vi "Periodic Tasks.vi"(8 "error in":errorcluster) -> ()   [LabVIEW 2020]
doc: "This VI runs in parallel to other tasks. It can contain as many user-defined periodic loops as you need. These can carry out PID or other sorts of timed response."
uses:
  <vilib>/Rock Robotics/WPI/Utilities/WPI_GetSetVariantRefNum.vi
  <vilib>/addons/control/pid/pid.llb/PID (DBL).vi
  <vilib>/addons/control/pid/NI_PID_pid.lvlib
panel:
  in  "output range":cluster{"output high":dbl, "output low":dbl}={"output high"=100.0, "output low"=-100.0} {"output low" format="%.2f"; "output high" format="%.2f"}
  in  "Output 2 PID gains":T1={"proportional gain (Kc)"=1.0, "integral time (Ti, min)"=0.01, "derivative time (Td, min)"=0.0} {"derivative time (Td, min)" format="%.3f"; "integral time (Ti, min)" format="%.3f"; "proportional gain (Kc)" format="%.3f"}
  in  "Output 2 RPM Setpoint":dbl
  in  "Output 2 Use PID":bool
  out "Shooter Stopped":bool
  in  "Output 2 Use limits":bool
  in  "Output 1 Use limits":bool
  out "Shooter Speed":dbl
  in  "Enabled 2":bool
  in  "Output 2":dbl(slide) scale=-1.0..1.0
  in  "Enabled":bool
  in  "Output":dbl(slide) scale=-1.0..1.0
  # "20 degrees angle,\n0.6 speed = 5 ft - 2400 rpm\n0.8 speed = 9 feet - 3000 rpm\nBattery at 11.8 volts"
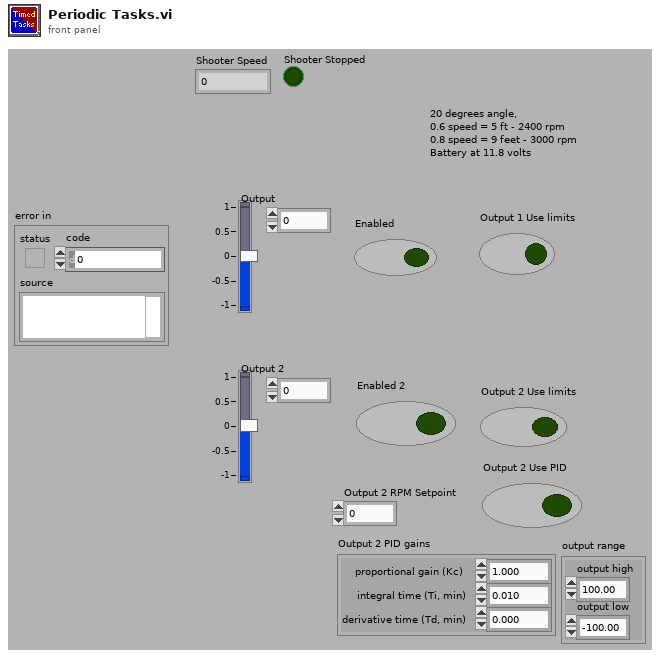
[diagram p1: front panel]
types:
  T1 = cluster{"proportional gain (Kc)":dbl, "integral time (Ti, min)":dbl, "derivative time (Td, min)":dbl}
  T2 = typedef "WPI_JoystickDevRef.ctl" = cluster{"Device":T3}
  T3 = typedef "WPI_JoystickDeviceEnum.ctl" = enum16{"USB 0", "USB 1", "USB 2", "USB 3", "USB 4", "USB 5"}
  T4 = typedef "WPI_MotorControlDeviceRef.ctl" = cluster{"DeviceStatus":errorcluster, "Type":T5, "PWM":cluster{"PWM Channel":T6, "DeadBand":T7}, "CAN":cluster{"Device Number":u8, "SetOutput VI Ref":variant, "GetOutput VI Ref":variant, "Enable VI Ref":variant, "Disable VI Ref":variant, "Data":variant}, "Invert":bool, "DIO PWM":cluster{"PWM \"Enable\" Channel":T6, "DIOChannel":T8, "PWM Rate":dbl}}
  T5 = typedef "WPI_MotorControlType.ctl" = enum16{"PWM", "CAN", "DIO PWM"}
  T6 = typedef "FPGA_DIOPWMChannel.ctl" = enum8{"PWM 0", "PWM 1", "PWM 2", "PWM 3", "PWM 4", "PWM 5", "PWM 6", "PWM 7", "PWM 8", "PWM 9", "PWM MXP 0", "PWM MXP 1", "PWM MXP 2", "PWM MXP 3", "PWM MXP 4", "PWM MXP 5", "PWM MXP 6", "PWM MXP 7", "PWM MXP 8", "PWM MXP 9", "Invalid"}
  T7 = typedef "WPI_PWMDeadband.ctl" = cluster{"Name":string, "maxPositivePwm":i32, "minPositivePwm":i32, "centerPwm":i32, "maxNegativePwm":i32, "minNegativePwm":i32, "angularRange":u16}
  T8 = typedef "FPGA_DIOChannel.ctl" = enum8{"DIO 0", "DIO 1", "DIO 2", "DIO 3", "DIO 4", "DIO 5", "DIO 6", "DIO 7", "DIO 8", "DIO 9", "DIO MXP 0", "DIO MXP 1", "DIO MXP 2", "DIO MXP 3", "DIO MXP 4", "DIO MXP 5", "DIO MXP 6", "DIO MXP 7", "DIO MXP 8", "DIO MXP 9", "DIO MXP 10", "DIO MXP 11", "DIO MXP 12", "DIO MXP 13", "DIO MXP 14", "DIO MXP 15", "SPI Port CS1", "SPI Port CS2", "SPI Port CS3", "SPI Port MISO", "SPI Port MOSI", "Invalid"}
  T9 = typedef "WPI_EncoderDevRef.ctl" = cluster{"DevStatus":errorcluster, "EncoderIndex":T10, "CounterIndex":T11, "DistancePerCount":dbl, "Decoding Type":T12}
  T10 = typedef "FPGA_EncoderIdx.ctl" = enum8{"Enc 0", "Enc 1", "Enc 2", "Enc 3", "Enc 4", "Enc 5", "Enc 6", "Enc 7", "Invalid"}
  T11 = typedef "FPGA_CounterCtrSystemIndex.ctl" = enum8{"Ctr 0", "Ctr 1", "Ctr 2", "Ctr 3", "Ctr 4", "Ctr 5", "Ctr 6", "Ctr 7", "Invalid"}
  T12 = typedef "WPI_EncoderType.ctl" = enum16{"1x", "2x", "4x"}
  T13 = typedef "WPI_SwitchDevRef.ctl" = cluster{"DevStatus":errorcluster, "DIO Channel":T8, "CntIndex":T11, "Normally Closed":bool}
  T14 = cluster{"JoystickDevRef":T2, "MotorControlDevRef":T4, "MotorControlDevRef":T4, "EncoderDevRef":T9, "SwitchDevRef":T13, "SwitchDevRef":T13}
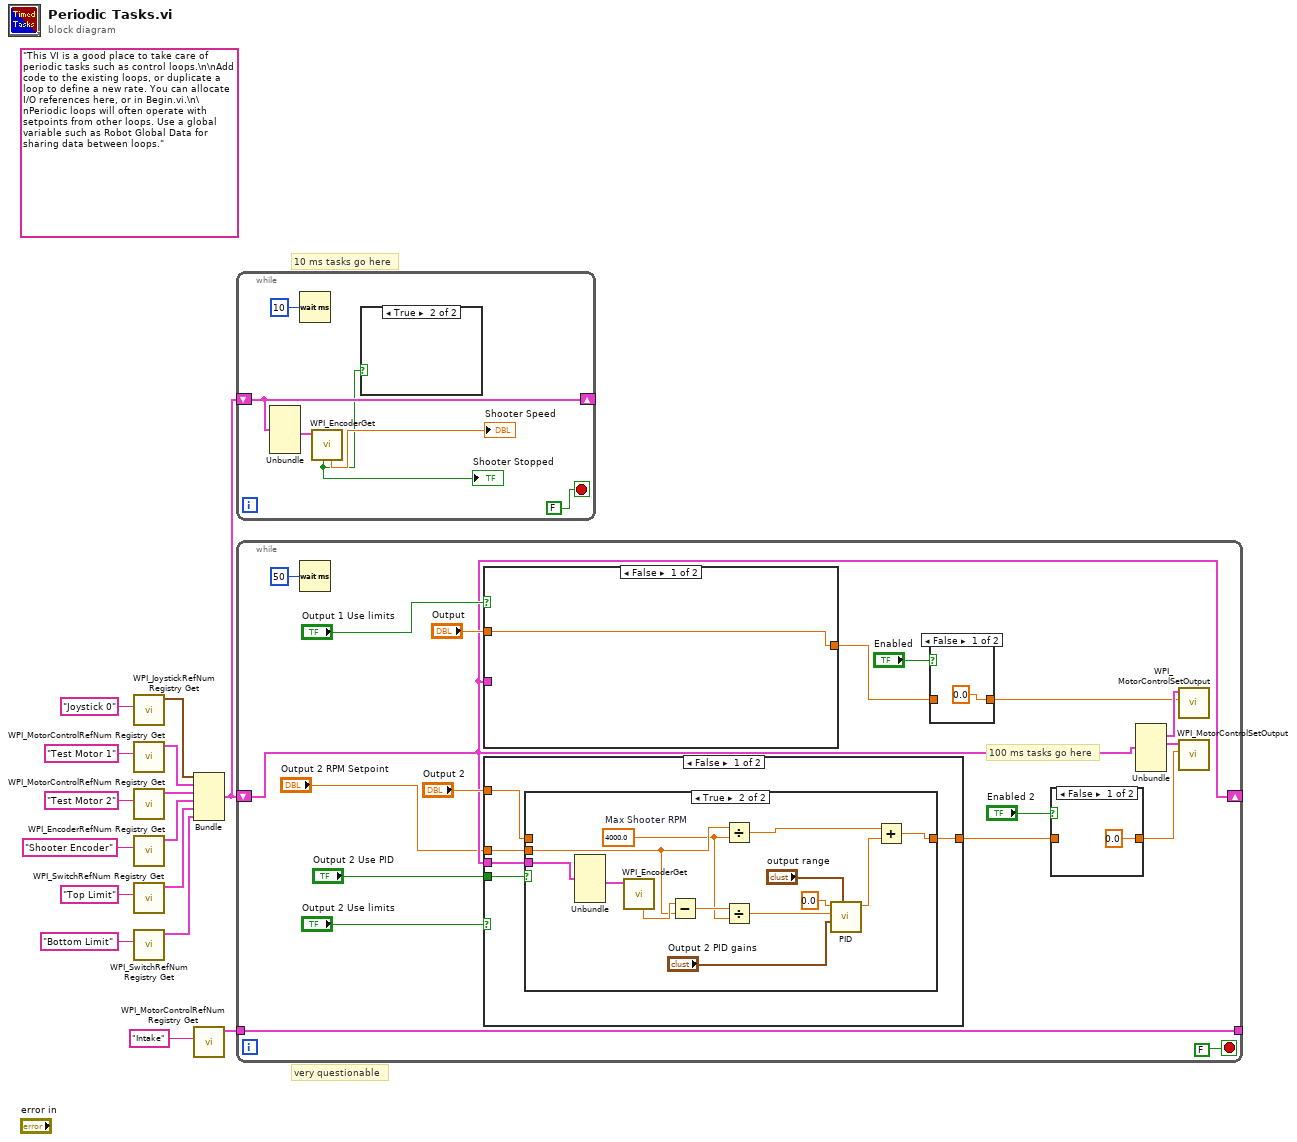
[diagram p0: block diagram]
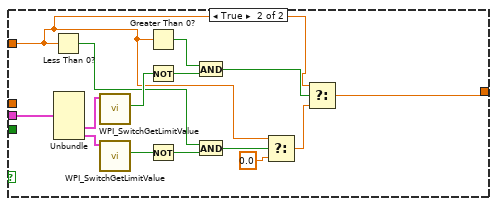
[diagram p5: hidden frame]
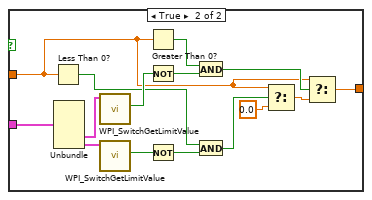
[diagram p6: hidden frame]
diagram:
  (unwired) "This VI is a good place to take care of periodic tasks such as control loops.\n\nAdd code to the existing loops, or duplicate a loop to define a new rate. You can allocate I/O references here, or in Begin.vi.\n\nPeriodic loops will often operate with setpoints from other loops. Use a global variable such as Robot Global Data for sharing data between loops."
  # "very questionable"
  # "10 ms tasks go here"
  n1 = call <vilib>:"WPI_JoystickRefNum Registry Get.vi"("refnum name"="Joystick 0") -> ("JoystickDevRef"=w14:T2)  [unwired: 1 in, 9 out]
  n2 = call <vilib>:"WPI_MotorControlRefNum Registry Get.vi"("refnum name"="Test Motor 1") -> ("MotorControlDevRef"=w11:T4)  [unwired: 9 in, 1 out]
  n3 = call <vilib>:"WPI_MotorControlRefNum Registry Get.vi"("refnum name"="Test Motor 2") -> ("MotorControlDevRef"=w9:T4)  [unwired: 9 in, 1 out]
  n4 = call <vilib>:"WPI_EncoderRefNum Registry Get.vi"("refnum name"="Shooter Encoder") -> ("EncoderDevRef"=w1:T9)  [unwired: 9 in, 1 out]
  n5 = call <vilib>:"WPI_SwitchRefNum Registry Get.vi"("refnum name"="Top Limit") -> ("SwitchDevRef"=w7:T13)  [unwired: 9 in, 1 out]
  n6 = call <vilib>:"WPI_SwitchRefNum Registry Get.vi"("refnum name"="Bottom Limit") -> ("SwitchDevRef"=w4:T13)  [unwired: 9 in, 1 out]
  n7 = Bundle("JoystickDevRef"=w14, "MotorControlDevRef"=w11, "MotorControlDevRef"=w9, "EncoderDevRef"=w1, "SwitchDevRef"=w7, "SwitchDevRef"=w4) -> (w13:T14)  [unwired: 1 out]
  n8 = call <vilib>:"WPI_MotorControlRefNum Registry Get.vi"("refnum name"="Intake") -> ("MotorControlDevRef"=w2:T4)  [unwired: 9 in, 1 out]
  n9 = while {
    shift-right: [w19] -> _
    shift-left: w13 -> [w19]
    stop <- FALSE stop-if-true
    n10 = Unbundle(w19) -> ("EncoderDevRef"=w17:T9)  [unwired: 5 out]
    n11 = Wait (ms)(milliseconds to wait=u32 10) -> ()  [unwired: 1 out]
    n12 = call <vilib>:"WPI_EncoderGet.vi"("EncoderDevRef"=w17) -> ("Rate"=→"Shooter Speed":dbl, "Stopped"=w16:bool)  [unwired: 5 in, 4 out]
    "Shooter Stopped" <- w16
    n13 = case shown="True" w16 {
      frame False {
      }
      frame True {
      }
    }
  }
  n14 = while {
    shift-right: [w33] -> _
    shift-left: w13 -> [w33]
    tunnel: [w25] -> _
    tunnel: w2 -> [w25]
    stop <- FALSE stop-if-true
    # "100 ms tasks go here"
    n15 = Wait (ms)(milliseconds to wait=u32 50) -> ()  [unwired: 1 out]
    n16 = case shown="False" "Output 1 Use limits" {
      tunnel: "Output" -> [w78 w80]
      tunnel: [w78 w87] -> w30
      tunnel: w33 -> [_ w93]
      frame False {
      }
      frame True {
        n17 = Less Than 0?(x=w80) -> (x < 0?=w86:bool)
        n18 = Unbundle(w93) -> ("SwitchDevRef"=w92:T13, "SwitchDevRef"=w81:T13)  [unwired: 4 out]
        n19 = call <vilib>:"WPI_SwitchGetLimitValue.vi"("SwitchDevRef"=w92) -> ("Switch Pressed"=w90:bool)  [unwired: 8 in, 2 out]
        n20 = call <vilib>:"WPI_SwitchGetLimitValue.vi"("SwitchDevRef"=w81) -> ("Switch Pressed"=w82:bool)  [unwired: 8 in, 2 out]
        n21 = Greater Than 0?(x=w80) -> (x > 0?=w91:bool)
        n22 = Not(x=w90) -> (.not. x?=w89:bool)
        n23 = Not(x=w82) -> (.not. x?=w85:bool)
        n24 = And(x=w91, y=w89) -> (x .and. y?=w88:bool)
        n25 = And(x=w86, y=w85) -> (x .and. y?=w84:bool)
        n26 = Select(t=w80, s=w84, f=0.0) -> (s? t:f=w79:dbl)
        n27 = Select(t=w80, s=w88, f=w79) -> (s? t:f=w87:dbl)
      }
    }
    n28 = case shown="False" "Output 2 Use limits" {
      tunnel: "Output 2" -> [w45 w64]
      tunnel: [w46 w71] -> w28
      tunnel: w33 -> [w44 w77]
      tunnel: "Output 2 Use PID" -> [w48 _]
      tunnel: "Output 2 RPM Setpoint" -> [w47 _]
      frame False {
        n29 = case shown="True" w48 {
          tunnel: w47 -> [_ w53]
          tunnel: [w49 w59] -> w46
          tunnel: w45 -> [w49 _]
          tunnel: w44 -> [_ w62]
          frame False {
          }
          frame True {
            w52 = 4000.0  # Max Shooter RPM
            n30 = Unbundle(w62) -> ("EncoderDevRef"=w61:T9)  [unwired: 5 out]
            n31 = call <vilib>:"WPI_EncoderGet.vi"("EncoderDevRef"=w61) -> ("Rate"=w56:dbl)  [unwired: 5 in, 5 out]
            n32 = Subtract(x=w56, y=w53) -> (x-y=w55:dbl)
            n33 = Divide(x=w53, y=w52) -> (x/y=w51:dbl)
            n34 = Divide(x=w55, y=w52) -> (x/y=w54:dbl)
            n35 = call-poly <vilib>:"PID.vi"("output range"="output range", "PID gains"="Output 2 PID gains", "process variable"=w54, "setpoint"=0.0) -> ("output"=w58:dbl)  [unwired: 6 in, 1 out]
            n36 = Add(x=w51, y=w58) -> (x+y=w59:dbl)
          }
        }
      }
      frame True {
        n37 = Less Than 0?(x=w64) -> (x < 0?=w70:bool)
        n38 = Unbundle(w77) -> ("SwitchDevRef"=w76:T13, "SwitchDevRef"=w65:T13)  [unwired: 4 out]
        n39 = call <vilib>:"WPI_SwitchGetLimitValue.vi"("SwitchDevRef"=w76) -> ("Switch Pressed"=w74:bool)  [unwired: 8 in, 2 out]
        n40 = call <vilib>:"WPI_SwitchGetLimitValue.vi"("SwitchDevRef"=w65) -> ("Switch Pressed"=w66:bool)  [unwired: 8 in, 2 out]
        n41 = Greater Than 0?(x=w64) -> (x > 0?=w75:bool)
        n42 = Not(x=w74) -> (.not. x?=w73:bool)
        n43 = Not(x=w66) -> (.not. x?=w69:bool)
        n44 = And(x=w75, y=w73) -> (x .and. y?=w72:bool)
        n45 = And(x=w70, y=w69) -> (x .and. y?=w68:bool)
        n46 = Select(t=w64, s=w68, f=0.0) -> (s? t:f=w63:dbl)
        n47 = Select(t=w64, s=w72, f=w63) -> (s? t:f=w71:dbl)
      }
    }
    n48 = case shown="False" "Enabled" {
      tunnel: w30 -> [_ w43]
      tunnel: [0.0 ("f") w43] -> w29
      frame False {
      }
      frame True {
      }
    }
    n49 = case shown="False" "Enabled 2" {
      tunnel: [0.0 ("Output") w41] -> w27
      tunnel: w28 -> [_ w41]
      frame False {
      }
      frame True {
      }
    }
    n50 = Unbundle(w33) -> ("MotorControlDevRef"=w37:T4, "MotorControlDevRef"=w36:T4)  [unwired: 4 out]
    n51 = call <vilib>:"WPI_MotorControlSetOutput.vi"("Output"=w29, "MotorControlDevRef"=w37) -> ()  [unwired: 7 in, 3 out]
    n52 = call <vilib>:"WPI_MotorControlSetOutput.vi"("Output"=w27, "MotorControlDevRef"=w36) -> ()  [unwired: 7 in, 3 out]
  }
